vi "Conditional Auto-Indexing Tunnel Example 01.vi"() -> ()   [LabVIEW 2019]
uses:
  user.lib/_OpenG.lib/array/array.llb/Conditional Auto-Indexing Tunnel (I32)__ogtk.vi
panel:
  out "Even Elements":i32[](array[numeric])
  in  "Array":i32[](array[numeric])=[1, 2, 3, 4, 5, 6, 7, 8]
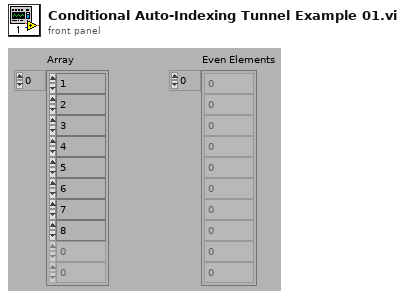
[diagram p1: front panel]
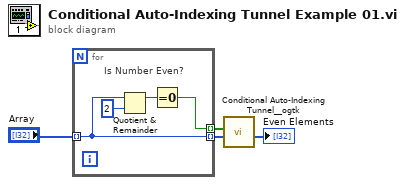
[diagram p0: block diagram]
diagram:
  n1 = for {
    tunnel: "Array" -> [w8] mode=indexing
    tunnel: [w5] -> w3 mode=indexing
    tunnel: [w8] -> w2 mode=indexing
    # "Is Number Even?"
    n2 = Quotient & Remainder(x=w8, y=2) -> (x-y*floor(x/y)=w6:i32)  [unwired: 1 out]
    n3 = Equal To 0?(x=w6) -> (x = 0?=w5:bool)
  }
  n4 = call-poly "Conditional Auto-Indexing Tunnel__ogtk.vi"("Array in"=w2, "Elements to keep"=w3) -> ("Filtered Array out"=→"Even Elements":i32[])  [unwired: 5 in]
